vi "Get Max ID OK Count.vi"(0 "connection reference":T1, 5 "Station No.":string, 11 "error in":errorcluster) -> (4 "connection reference out":T1, 6 "MAX BREAKDOWN ID":i32, 8 "PRODUCTION COUNT":i32, 10 "Table Name":string, 15 "error out":errorcluster)   [LabVIEW 2017]
uses:
  <vilib>/addons/database/Connection.llb/Conn ObjectReference.ctl
  <vilib>/addons/database/NI_Database_API.lvlib
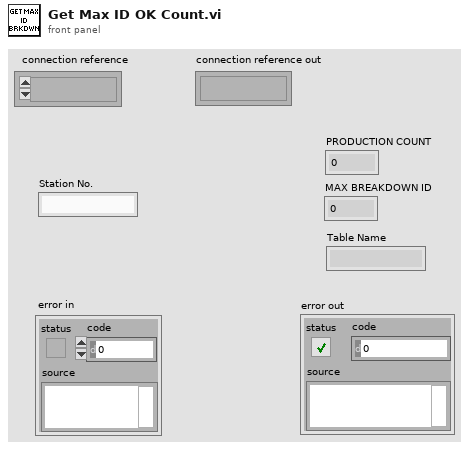
[diagram p1: front panel]
types:
  T1 = typedef "NI_Database_API.lvlib/Conn ObjectReference.ctl" = refnum<k1>
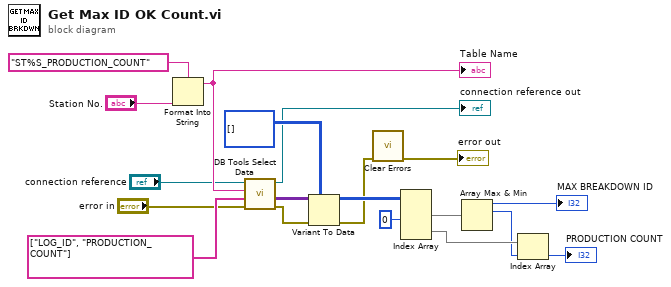
[diagram p0: block diagram]
diagram:
  n1 = Format Into String(format string="ST%S_PRODUCTION_COUNT" ("SQL query"), "Station No.") -> (resulting string=w6:string)  [unwired: 2 in, 1 out]
  "Table Name" <- w6
  n2 = call <vilib>:"DB Tools Select Data.vi"("error in (no error)"="error in", "columns"=string[] ["LOG_ID", "PRODUCTION_COUNT"], "table"=w6, "connection reference"="connection reference") -> ("error out"=w16:errorcluster, "data"=w17:variant[][], "connection reference out"=→"connection reference out":T1)  [unwired: 2 in]
  n3 = Variant To Data(error in=w16, type=i32[][] [] ("columns"), Variant=w17) -> (data=w15:i32[][], error out=w3:errorcluster)
  n4 = call <vilib>:"Clear Errors.vi"("error in (no error)"=w3) -> ("error out"=→"error out":errorcluster)  [unwired: 5 in, 1 out]
  n5 = Index Array(array=w15, index (col) #1=0 ("disabled index (col)")) -> (element #1=w14:i32[], element #2=w11:i32[])  [unwired: 3 in]
  n6 = Array Max & Min(array=w14) -> (max value=→"MAX BREAKDOWN ID":i32, max index (indices)=w10:i32)  [unwired: 2 out]
  n7 = Index Array(array=w11, index=w10) -> (element=→"PRODUCTION COUNT":i32)
